vi "Template Constructor.vi"(8 "error in (no error)":errorcluster) -> (0 "error out":errorcluster, 3 "Mock Class Generator out":refnum<class>)   [LabVIEW 2020, in "Templates.lvlib"]
uses:
  Templates.lvlib
  Framework/Responsive Mock/Responsive Mock.lvclass
  C:/git/astemes-lmock/source/Framework/Mock/Mockito.lvclass
  C:/git/astemes-lmock/source/Framework/Responsive Mock/Responsive Mock.lvclass
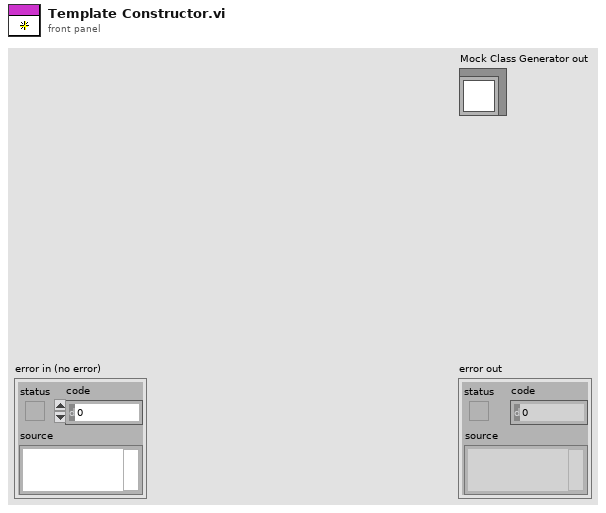
[diagram p1: front panel]
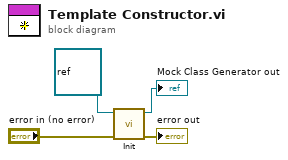
[diagram p0: block diagram]
diagram:
  n1 = call-dynamic "Init.vi"("error in (no error)"="error in (no error)", "Mock In"=refnum<class> refnum ("Mock in")) -> ("error out"=→"error out":errorcluster, "Mock Out"=→"Mock Class Generator out":refnum<class "Responsive Mock.lvclass">)  [unwired: 8 in]
